vi "Abort Notification to All.vi"(8 "error in (no error)":errorcluster, 11 "Simple Map Notifier Controller in":refnum<class "Map Notifier Controller.lvclass">) -> (0 "error out":errorcluster, 3 "Simple Map Notifier Controller out":refnum<class "Map Notifier Controller.lvclass">)   [LabVIEW 2024, in "Map Notifier Controller.lvclass"]
uses:
  Map Notifier Controller.lvclass
  Map Notifier Controller.lvclass/Map Notifier Controller.ctl
  Ancestor Class/Actor Assistant/Notifier/Notifier.lvclass
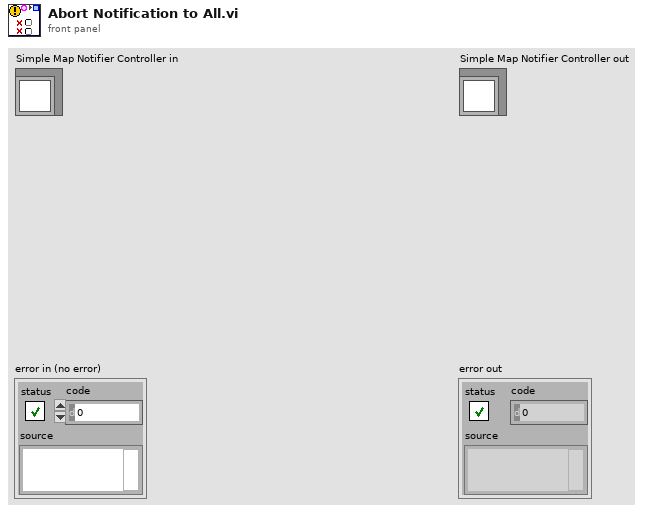
[diagram p1: front panel]
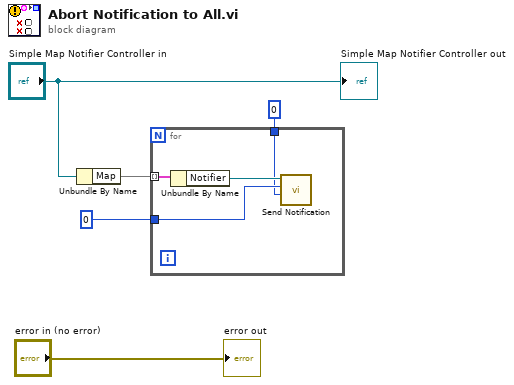
[diagram p0: block diagram]
diagram:
  n1 = Unbundle By Name("Simple Map Notifier Controller in") -> ("Map"=w4:map{i64, refnum<class "Notifier.lvclass">})
  n2 = for {
    tunnel: w4 -> [w9] mode=indexing
    tunnel: i64 0 ("Timeout") -> [w7]
    tunnel: 0 ("Timeout") -> [w6]
    n3 = Unbundle By Name(w9) -> ("Notifier"=w8:refnum<class "Notifier.lvclass">)
    n4 = call-dynamic "Send Notification.vi"("Timeout"=w6, "Notification"=w7, "Notifier in"=w8) -> ()  [unwired: 6 in, 3 out]
  }
  "error out" <- "error in (no error)"
  "Simple Map Notifier Controller out" <- "Simple Map Notifier Controller in"
